vi "dual camera load displacement.vi"() -> ()   [LabVIEW 2013]
uses:
  <vilib>/userdefined/High Color/IMAQdx.ctl
  <vilib>/vision/driver/IMAQdx.llb/IMAQdx Buffer Number Mode.ctl
  <vilib>/Analysis/baseanly.llb/Mean (DBL).vi
  Instance           1 30Saved   Shear-C273-with-Unload .vi
  Instance           4 30Saved   Shear-C273-with-Unload .vi
  <vilib>/vision/driver/NI_Vision_Acquisition_Software.lvlib
  <resource>/objmgr/imaqdx.rc
  <vilib>/Analysis/NI_AALBase.lvlib
panel:
  in  "Shutter 3":dbl(slide)=20.0 min=0.0 max=4095.0 step=1.0 scale=4.095..4095.0 scale format="%#.0f"
  in  "Brightness 3":dbl(slide)=200.0 min=0.0 max=255.0 step=1.0 scale=0.0..255.0
  in  "Gain 3":dbl(slide)=702.0 min=350.0 max=1000.0 step=1.0 scale=350.0..1000.0
  out "Boolean 2":bool
  in  "Image Sampling Frequency (ms) 2":u32=100
  in  "Save nth image 2":i32=10
  in  "Capture Current Image 2":bool
  out "Diagonal":T1(plugin-control)
  in  "Video Mode Top 2":u32(ring)=47 items=["320x240 Color"=4, "640x480 Mono8"=9, "640x480 Mono16"=19, "640x480 Color"=14, "800x600 Mono8"=21, "800x600 Mono16"=27, "800x600 Color"=24, "1024x768 Mono8"=30, "1024x768 Mono16"=36, "1024x768 Color"=33, "1280x960 Mono8"=40, "1280x960 Mono16"=46, "1280x960 Color"=43, "1388x1038 Color"=47, "1388x1038 Mono"=48]
  in  "Session In Top View 2":T2="cam1"
  out "Side":T1(plugin-control)
  out "x-y":u32
  out "Boolean":bool
  in  "Begin Loading 2":bool
  in  "Shutter":dbl(slide)=20.0 min=0.0 max=4095.0 step=1.0 scale=4.095..4095.0 scale format="%#.0f"
  in  "Brightness":dbl(slide)=200.0 min=0.0 max=255.0 step=1.0 scale=0.0..255.0
  in  "Gain":dbl(slide)=702.0 min=350.0 max=1000.0 step=1.0 scale=350.0..1000.0
  in  "Video Mode Top":u32(ring)=47 items=["320x240 Color"=4, "640x480 Mono8"=9, "640x480 Mono16"=19, "640x480 Color"=14, "800x600 Mono8"=21, "800x600 Mono16"=27, "800x600 Color"=24, "1024x768 Mono8"=30, "1024x768 Mono16"=36, "1024x768 Color"=33, "1280x960 Mono8"=40, "1280x960 Mono16"=46, "1280x960 Color"=43, "1388x1038 Color"=47, "1388x1038 Mono"=48]
  in  "Session In Top View":T2="cam1"
  in  "Image Sampling Frequency (ms)":u32=100
  in  "Stop 2":bool
  in  "Save nth image":i32=10
  in  "Capture Current Image":bool
  in  "Begin Loading":bool
  out "Displacement (mm)":dbl
  in  "Pause":bool
  out "Crosshead Displacement":cluster{dbl[], dbl[]}(graph)
  in  "Unload Velocity":dbl=500.0
  in  "Unload":bool
  in  "Load Cell\nSelection":enum16{"300lb", "5lb", "50lb", "100lb"}(ring)=enum."50lb"
  in  "Distance to Travel (microns) \nup is positive":dbl=250000.0
  in  "Velocity (microns/sec)":dbl=5.0
  in  "Filename":string="test2"
  in  "Storage Directory":path=path "C:/Documents and Settings/AMS_Beckman/My Documents/Users_2010_2011/Jason_Patrick"
  in  "Material":string
  in  "Stop":bool
  # "Edge Parameters"
  # "Top View Camera"
types:
  T1 = typedef "IMAQ Image.ctl" = refnum<image>
  T2 = typedef "IMAQdx.ctl" = refnum<k21>
  T3 = typedef "Image Type" = u32
  T4 = enum16{"open", "open or create", "create or replace", "create", "open (read only)"}
  T5 = typedef "NI_Vision_Acquisition_Software.lvlib/IMAQdx Buffer Number Mode.ctl" = enum32{"Next", "Last", "Buffer Number"}
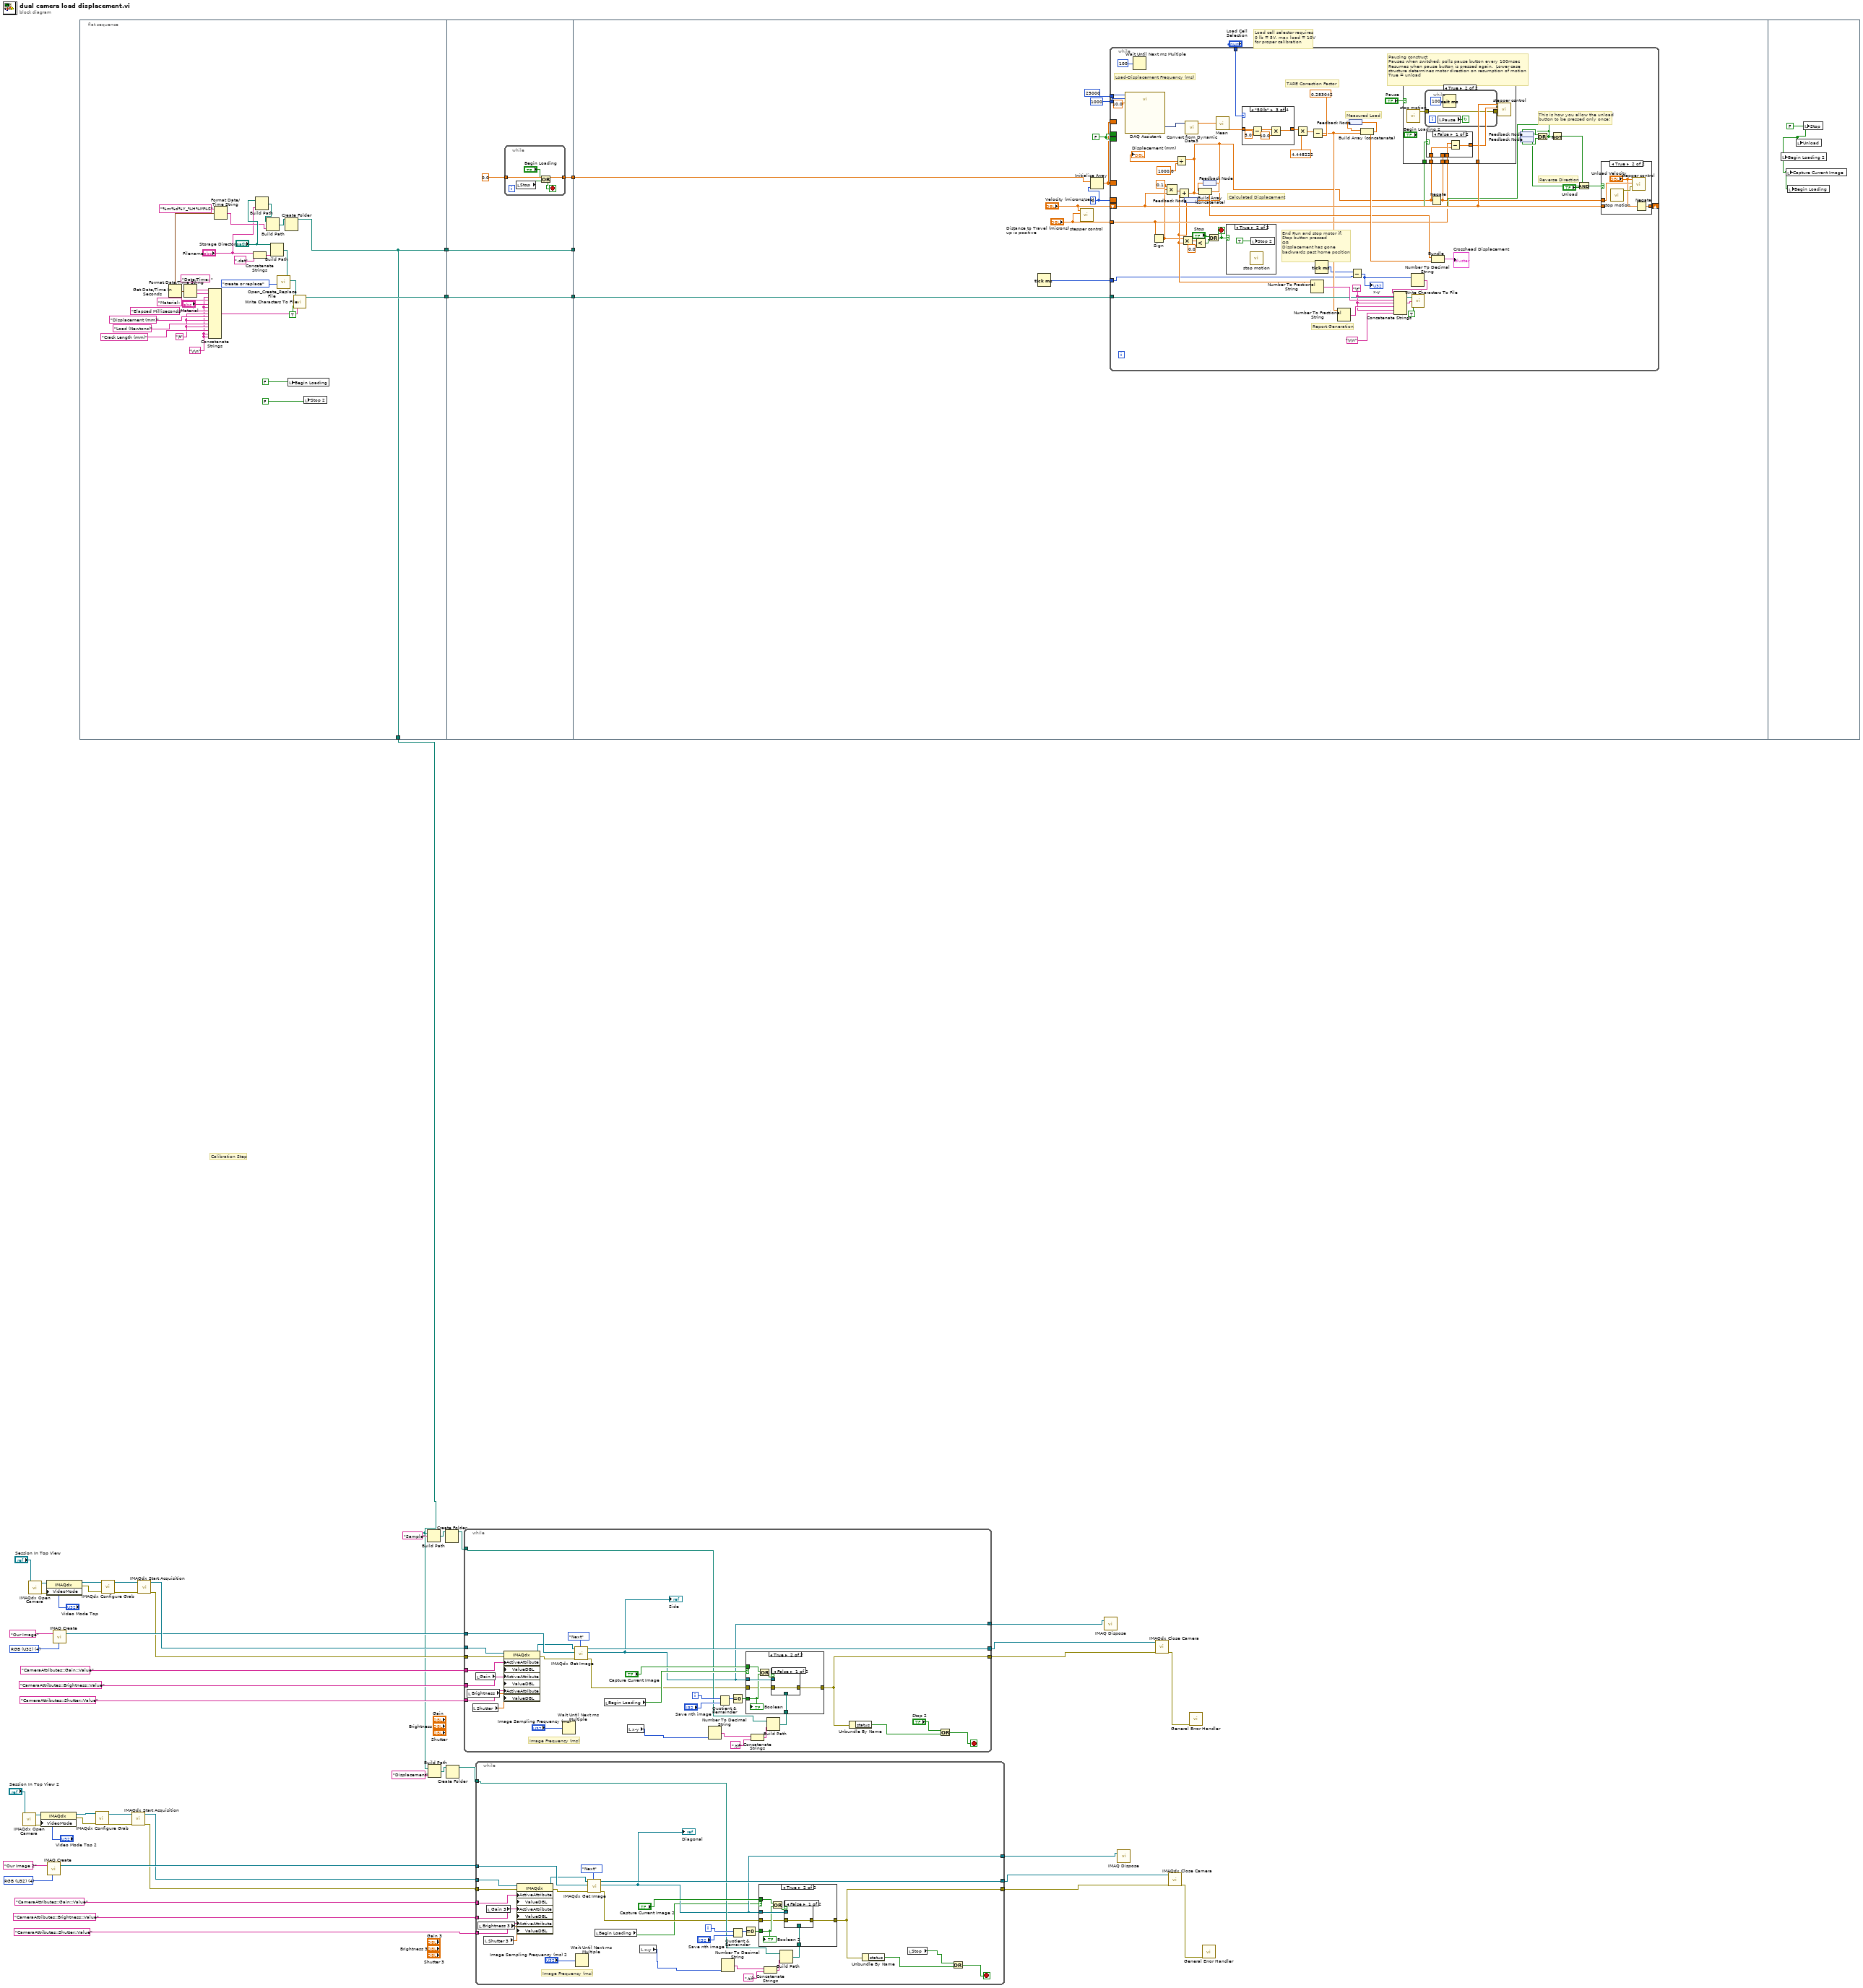
[diagram p0: block diagram]
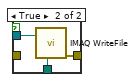
[diagram p3: hidden frame]
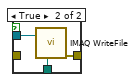
[diagram p5: hidden frame]
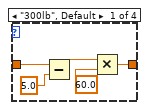
[diagram p10: hidden frame]
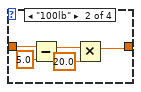
[diagram p11: hidden frame]
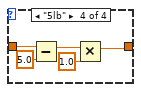
[diagram p12: hidden frame]
diagram:
  w23 = T3 4 items=["Grayscale (U8)", "Grayscale (I16)", "Grayscale (SGL)", "Complex (CSG)", "RGB (U32)", "HSL (U32)", "RGB (U64)"] ("Image Type")
  w43 = T3 4 items=["Grayscale (U8)", "Grayscale (I16)", "Grayscale (SGL)", "Complex (CSG)", "RGB (U32)", "HSL (U32)", "RGB (U64)"] ("Image Type")
  # "Calibration Step"
  n1 = call <vilib>:"IMAQdx Open Camera.vi"("Session In"="Session In Top View 2") -> ("error out"=w21:errorcluster, "Session Out"=w22:T2)  [unwired: 9 in]
  n2 = call <vilib>:"IMAQdx Open Camera.vi"("Session In"="Session In Top View") -> ("error out"=w41:errorcluster, "Session Out"=w42:T2)  [unwired: 9 in]
  n3 = property class="IMAQdx"(reference=w22, error in=w21, "VideoMode"="Video Mode Top 2") -> (reference out=w19:T2, error out=w20:errorcluster)
  n4 = property class="IMAQdx"(reference=w42, error in=w41, "VideoMode"="Video Mode Top") -> (reference out=w39:T2, error out=w40:errorcluster)
  n5 = call "IMAQ Create"("Image Name"="Our Image 2", "Image Type"=w23) -> ("New Image"=w10:T1)  [unwired: 3 in, 1 out]
  n6 = call "IMAQ Create"("Image Name"="Our Image", "Image Type"=w43) -> ("New Image"=w34:T1)  [unwired: 3 in, 1 out]
  n7 = flat-sequence {
    tunnel: [w71] -> w52
    tunnel: [w65] -> w50
    tunnel: [w65] -> w2
    tunnel: w52 -> [w84]
    tunnel: [w84] -> w51
    tunnel: w50 -> [w83]
    tunnel: [w83] -> w49
    tunnel: [w81] -> w48
    tunnel: w51 -> [w94]
    tunnel: w49 -> [_]
    tunnel: w48 -> [w90]
    frame #0 {
      w58 = "\t"
      w57 = "\r\n"
      n8 = Get Date/Time In Seconds() -> (seconds since 1Jan1904=w67:timestamp)
      n9 = Format Date/Time String(seconds (now)=w67) -> (date/time string=w73:string)  [unwired: 2 in]
      n10 = Concatenate Strings("Date/Time: ", w73, w57, "Material:  ", "Material", w57, "Elapsed Milliseconds" ("string"), w58, "Displacement (mm)" ("string"), w58, "Load (Newtons)" ("string"), w58, "Crack Length (mm)" ("string"), w57, w57) -> (w75:string)
      n11 = Format Date/Time String(time format string (%c)="%m%d%Y_%H%M%S", seconds (now)=w67) -> (date/time string=w54:string)  [unwired: 1 in]
      n12 = Concatenate Strings("Filename", ".dat") -> (w77:string)
      n13 = Build Path(base path="Storage Directory", name or relative path="Filename") -> (appended path=w55:path)
      n14 = Build Path(base path=w55, name or relative path=w54) -> (appended path=w69:path)
      n15 = Build Path(base path="Storage Directory", name or relative path=w77) -> (appended path=w70:path)
      n16 = call <vilib>:"Open_Create_Replace File.vi"("function (open:0)"=T4."create or replace", "file path"=w70) -> ("new file path"=w79:path)  [unwired: 6 in, 3 out]
      n17 = Create Folder(path (use dialog)=w69) -> (created path=w65:path)  [unwired: 2 in, 2 out]
      n18 = local write "Begin Loading"(FALSE ("Begin Loading")) -> ()
      n19 = call <vilib>:"Write Characters To File.vi"("append to file? (new file:F)"=TRUE, "character string"=w75, "file path (dialog if empty)"=w79) -> ("new file path (Not A Path if cancelled)"=w71:path)  [unwired: 2 in]
      n20 = local write "Stop 2"(FALSE ("Stop 2")) -> ()
    }
    frame #1 {
      n21 = while {
        tunnel: [w88] -> w81
        tunnel: 0.0 ("element") -> [w88]
        stop <- w86 stop-if-true
        n22 = local read "Stop"() -> (w85:bool)
        n23 = Or(x="Begin Loading", y=w85) -> (x .or. y?=w86:bool)
      }
    }
    frame #2 {
      w99 = FALSE
      w98 = 0 ("dimension size")
      # "Load cell selector requires\n0 lb = 5V, max load = 10V\nfor proper calibration"
      n24 = Tick Count (ms)() -> (millisecond timer value=w89:u32)
      n25 = call "stepper control.vi"("Distance to Travel (microns) \nup  is positive"="Distance to Travel (microns) \nup is positive", "Velocity (microns/sec)"="Velocity (microns/sec)") -> ()  [unwired: 9 in, 1 out]
      n26 = Initialize Array(w90, w98) -> (w97:dbl[])
      n27 = while {
        tunnel: "Load Cell\nSelection" -> [w150]
        tunnel: w94 -> [w140]
        shift-right: [w139] -> _
        shift-left: "Velocity (microns/sec)" -> [w124]
        tunnel: "Distance to Travel (microns) \nup is positive" -> [w121]
        border: w97 -> [_]
        border: w98 -> [_]
        border: w97 -> [_]
        border: w99 -> [_]
        border: w99 -> [_]
        tunnel: 25000 ("Sampling Rate") -> [w115]
        tunnel: 1000 ("Sampling Rate") -> [w114]
        tunnel: w89 -> [w103]
        stop <- w138 stop-if-true
        w105 = "\t"
        # "Load-Displacement Frequency (ms)"
        # "TARE Correction Factor"
        # "Pausing construct\nPauses when switched; polls pause button every 100msec\nResumes when pause button is pressed again.  Lower case\nstructure determines motor direction on resumption of motion\nTrue = unload"
        # "This is how you allow the unload\nbutton to be pressed only once!"
        # "Reverse Direction"
        # "Calculated Displacement"
        # "Measured Load"
        # "End Run and stop motor if:\nStop button pressed\nOR\nDisplacement has gone \nbackwards past home position"
        # "Report Generation"
        n28 = call "DAQ Assistant"("rate"=w115, "number of samples"=w114, "timeout (s)"=10.0 ("timeout (sec)")) -> ("data"=w116:dynamicdata)  [unwired: 14 in, 2 out]
        n29 = Wait Until Next ms Multiple(millisecond multiple=100 ("Loop Timing")) -> ()  [unwired: 1 out]
        n30 = Sign(1:w121) -> (0:w118:dbl)
        n31 = Compound Arithmetic op=MULTIPLY(0.1 ("x"), w118, w124) -> (w135:dbl)
        n32 = feedback #1() -> (w119:dbl)
        n33 = Add(x=w135, y=w119) -> (x+y=w108:dbl)
        n34 = Divide(x=w108, y=1000.0 ("timeout (sec)")) -> (x/y=→"Displacement (mm)":dbl)
        n35 = Multiply(x=w118, y=w119) -> (x*y=w120:dbl)
        n36 = feedback-in #1(w108) -> ()
        n37 = call "Convert from Dynamic Data3"("Dynamic Data Type"=w116) -> ("Array"=w113:dbl[])  [unwired: 3 in]
        n38 = Less?(x=w120, y=0.0) -> (x < y?=w137:bool)
        n39 = feedback #2() -> (w146:dbl[])
        n40 = Build Array (concatenate)(w146, w108) -> (w126:dbl[])
        n41 = feedback-in #2(w126) -> ()
        n42 = Or(x="Stop", y=w137) -> (x .or. y?=w138:bool)
        n43 = call-poly <vilib>:"Mean.vi"("X"=w113) -> ("mean"=w112:dbl)  [unwired: 1 out]
        n44 = case shown="True" w138 {
          frame False {
          }
          frame True {
            n45 = call "stop motion.vi"() -> ()  [unwired: 11 in, 1 out]
            n46 = local write "Stop 2"(TRUE ("Stop 2")) -> ()
          }
        }
        n47 = case shown="\"50lb\"" w150 {
          tunnel: w112 -> [w175 w179 w187 w192]
          tunnel: [w177 w178 w186 w191] -> w148
          frame "300lb", Default {
            n48 = Subtract(x=w175, y=5.0) -> (x-y=w173:dbl)
            n49 = Multiply(x=w173, y=60.0) -> (x*y=w177:dbl)
          }
          frame "100lb" {
            n50 = Subtract(x=w179, y=5.0) -> (x-y=w181:dbl)
            n51 = Multiply(x=w181, y=20.0) -> (x*y=w178:dbl)
          }
          frame "50lb" {
            n52 = Subtract(x=w187, y=5.0) -> (x-y=w184:dbl)
            n53 = Multiply(x=w184, y=10.0) -> (x*y=w186:dbl)
          }
          frame "5lb" {
            n54 = Subtract(x=w192, y=5.0) -> (x-y=w189:dbl)
            n55 = Multiply(x=w189, y=1.0) -> (x*y=w191:dbl)
          }
        }
        n56 = Multiply(x=w148, y=4.448222) -> (x*y=w111:dbl)
        n57 = Number To Fractional String(number=w119) -> (F-format string=w142:string)  [unwired: 3 in]
        n58 = Subtract(x=w111, y=0.283042) -> (x-y=w109:dbl)
        n59 = Tick Count (ms)() -> (millisecond timer value=w102:u32)
        n60 = Number To Fractional String(number=w109) -> (F-format string=w141:string)  [unwired: 3 in]
        n61 = feedback #3() -> (w147:dbl[])
        n62 = Subtract(x=w102, y=w103) -> (x-y=w101:u32)
        "x-y" <- w101
        n63 = Build Array (concatenate)(w147, w109) -> (w127:dbl[])
        n64 = feedback-in #3(w127) -> ()
        n65 = Number To Decimal String(number=w101) -> (decimal integer string=w104:string)  [unwired: 1 in]
        n66 = Concatenate Strings(w104, w105, w142, w105, w141, w105, "\r\n") -> (w144:string)
        n67 = call <vilib>:"Write Characters To File.vi"("append to file? (new file:F)"=TRUE, "character string"=w144, "file path (dialog if empty)"=w140) -> ()  [unwired: 2 in, 1 out]
        n68 = Negate(x=w108) -> (-x=w122:dbl)
        n69 = Bundle(w126, w127) -> (→"Crosshead Displacement":cluster{dbl[], dbl[]})  [unwired: 1 in]
        n70 = feedback #4() -> (w134:bool)
        n71 = feedback #5() -> (w132:bool)
        n72 = Or(x=w134, y=w132) -> (x .or. y?=w123:bool)
        n73 = case shown="True" "Pause" {
          tunnel: w124 -> [_ w157]
          tunnel: w123 -> [_ w156]
          tunnel: w122 -> [_ w155]
          tunnel: w121 -> [_ w154]
          tunnel: w108 -> [_ w152]
          frame False {
          }
          frame True {
            n74 = call "stop motion.vi"() -> ("error out"=w159:errorcluster)  [unwired: 11 in]
            n75 = while {
              tunnel: [w164] -> w158
              tunnel: w159 -> [w164]
              stop <- w166 continue-if-true
              n76 = local read "Pause"() -> (w166:bool)
              n77 = Wait (ms)(milliseconds to wait=100 ("Loop Timing")) -> ()  [unwired: 1 out]
            }
            n78 = case shown="False" w156 {
              tunnel: w155 -> [_ w163]
              tunnel: w154 -> [w161 _]
              tunnel: [w162 w163] -> w153
              tunnel: w152 -> [w160 _]
              frame False {
                n79 = Subtract(x=w161, y=w160) -> (x-y=w162:dbl)
              }
              frame True {
              }
            }
            n80 = call "stepper control.vi"("error in (no error)"=w158, "Distance to Travel (microns) \nup  is positive"=w153, "Velocity (microns/sec)"=w157) -> ()  [unwired: 8 in, 1 out]
          }
        }
        n81 = feedback-in #4(w123) -> ()
        n82 = Not(x=w123) -> (.not. x?=w133:bool)
        n83 = And(x=w133, y="Unload") -> (x .and. y?=w130:bool)
        n84 = feedback-in #5(w130) -> ()
        n85 = case shown="True" w130 {
          tunnel: w122 -> [_ w170]
          tunnel: [w167 w169] -> w139
          tunnel: w124 -> [w167 _]
          frame False {
          }
          frame True {
            n86 = call "stop motion.vi"() -> ("error out"=w171:errorcluster)  [unwired: 11 in]
            n87 = call "stepper control.vi"("error in (no error)"=w171, "Distance to Travel (microns) \nup  is positive"=w170, "Velocity (microns/sec)"="Unload Velocity") -> ()  [unwired: 8 in, 1 out]
            n88 = Negate(x="Unload Velocity") -> (-x=w169:dbl)
          }
        }
      }
    }
    frame #3 {
      w193 = FALSE ("Stop")
      n89 = local write "Begin Loading 2"(w193) -> ()
      n90 = local write "Capture Current Image"(w193) -> ()
      n91 = local write "Begin Loading"(w193) -> ()
      n92 = local write "Unload"(w193) -> ()
      n93 = local write "Stop"(w193) -> ()
    }
  }
  n94 = call <vilib>:"IMAQdx Configure Grab.vi"("error in"=w20, "Session In"=w19) -> ("error out"=w17:errorcluster, "Session Out"=w18:T2)  [unwired: 8 in]
  n95 = call <vilib>:"IMAQdx Configure Grab.vi"("error in"=w40, "Session In"=w39) -> ("error out"=w37:errorcluster, "Session Out"=w38:T2)  [unwired: 8 in]
  n96 = call <vilib>:"IMAQdx Start Acquisition.vi"("error in"=w17, "Session In"=w18) -> ("error out"=w8:errorcluster, "Session Out"=w9:T2)  [unwired: 8 in]
  n97 = call <vilib>:"IMAQdx Start Acquisition.vi"("error in"=w37, "Session In"=w38) -> ("error out"=w25:errorcluster, "Session Out"=w35:T2)  [unwired: 8 in]
  n98 = Build Path(base path=w2, name or relative path="Sample") -> (appended path=w27:path)
  n99 = Build Path(base path=w2, name or relative path="Displacement") -> (appended path=w4:path)
  n100 = Create Folder(path (use dialog)=w27) -> (created path=w26:path)  [unwired: 2 in, 2 out]
  n101 = Create Folder(path (use dialog)=w4) -> (created path=w3:path)  [unwired: 2 in, 2 out]
  n102 = while {
    tunnel: w34 -> [w219]
    tunnel: "CameraAttributes::Gain::Value" ("ActiveAttribute") -> [w225]
    tunnel: "CameraAttributes::Brightness::Value" ("ActiveAttribute") -> [w224]
    tunnel: "CameraAttributes::Shutter::Value" ("ActiveAttribute") -> [w223]
    tunnel: [w213] -> w47
    tunnel: w25 -> [w217]
    tunnel: [w210] -> w46
    tunnel: w35 -> [w214]
    tunnel: [w194] -> w29
    tunnel: w26 -> [w196]
    i -> [w206]
    stop <- w209 stop-if-true
    # "Image Frequency (ms)"
    n103 = local read "Brightness"() -> (w221:dbl)
    n104 = local read "Shutter"() -> (w220:dbl)
    n105 = local read "Gain"() -> (w222:dbl)
    n106 = property class="IMAQdx"(reference=w214, error in=w217, "ActiveAttribute"=w225, "ValueDBL"=w222, "ActiveAttribute"=w224, "ValueDBL"=w221, "ActiveAttribute"=w223, "ValueDBL"=w220) -> (reference out=w216:T2, error out=w215:errorcluster)
    n107 = Wait Until Next ms Multiple(millisecond multiple="Image Sampling Frequency (ms)") -> ()  [unwired: 1 out]
    n108 = call <vilib>:"IMAQdx Get Image.vi"("Buffer Number Mode (Next)"=IMAQdx_Buffer_Number_Mode."Next", "error in"=w215, "Image In"=w219, "Session In"=w216) -> ("error out"=w195:errorcluster, "Image Out"=w194:T1, "Session Out"=w213:T2)  [unwired: 4 in, 1 out]
    "Side" <- w194
    n109 = local read "Begin Loading"() -> (w202:bool)
    n110 = local read "x-y"() -> (w199:u32)
    n111 = Number To Decimal String(number=w199) -> (decimal integer string=w197:string)  [unwired: 1 in]
    n112 = Quotient & Remainder(x=w206, y="Save nth image") -> (x-y*floor(x/y)=w204:i32)  [unwired: 1 out]
    n113 = Equal To 0?(x=w204) -> (x = 0?=w203:bool)
    n114 = Concatenate Strings(w197, ".tif") -> (w211:string)
    n115 = Build Path(base path=w196, name or relative path=w211) -> (appended path=w212:path)
    n116 = case shown="True" w202 {
      tunnel: w194 -> [_ w233]
      tunnel: w212 -> [_ w231]
      tunnel: [w226 w232] -> w210
      tunnel: "Capture Current Image" -> [_ w229]
      tunnel: w203 -> [_ w228]
      tunnel: w195 -> [w226 w227]
      frame False {
      }
      frame True {
        n117 = Or(x=w229, y=w228) -> (x .or. y?=w230:bool)
        n118 = case shown="False" w230 {
          tunnel: w233 -> [_ w237]
          tunnel: [w234 w236] -> w232
          tunnel: w231 -> [_ w235]
          tunnel: w227 -> [w234 _]
          frame False {
          }
          frame True {
            n119 = call "IMAQ WriteFile"("File Path"=w235, "Image"=w237) -> ("error out"=w236:errorcluster)  [unwired: 6 in]
          }
        }
        "Boolean" <- w228
      }
    }
    n120 = Unbundle By Name(w210) -> ("status"=w208:bool)
    n121 = Or(x="Stop 2", y=w208) -> (x .or. y?=w209:bool)
  }
  n122 = while {
    tunnel: w10 -> [w263]
    tunnel: "CameraAttributes::Gain::Value" ("ActiveAttribute") -> [w269]
    tunnel: "CameraAttributes::Brightness::Value" ("ActiveAttribute") -> [w268]
    tunnel: "CameraAttributes::Shutter::Value" ("ActiveAttribute") -> [w267]
    tunnel: [w257] -> w14
    tunnel: w8 -> [w261]
    tunnel: [w254] -> w13
    tunnel: w9 -> [w258]
    tunnel: [w241] -> w11
    tunnel: w3 -> [w243]
    i -> [w250]
    stop <- w253 stop-if-true
    # "Image Frequency (ms)"
    n123 = local read "Brightness 3"() -> (w265:dbl)
    n124 = local read "Shutter 3"() -> (w264:dbl)
    n125 = local read "Gain 3"() -> (w266:dbl)
    n126 = property class="IMAQdx"(reference=w258, error in=w261, "ActiveAttribute"=w269, "ValueDBL"=w266, "ActiveAttribute"=w268, "ValueDBL"=w265, "ActiveAttribute"=w267, "ValueDBL"=w264) -> (reference out=w260:T2, error out=w259:errorcluster)
    n127 = Wait Until Next ms Multiple(millisecond multiple="Image Sampling Frequency (ms) 2") -> ()  [unwired: 1 out]
    n128 = call <vilib>:"IMAQdx Get Image.vi"("Buffer Number Mode (Next)"=IMAQdx_Buffer_Number_Mode."Next", "error in"=w259, "Image In"=w263, "Session In"=w260) -> ("error out"=w242:errorcluster, "Image Out"=w241:T1, "Session Out"=w257:T2)  [unwired: 4 in, 1 out]
    "Diagonal" <- w241
    n129 = local read "Begin Loading"() -> (w239:bool)
    n130 = local read "x-y"() -> (w238:u32)
    n131 = Number To Decimal String(number=w238) -> (decimal integer string=w244:string)  [unwired: 1 in]
    n132 = Quotient & Remainder(x=w250, y="Save nth image 2") -> (x-y*floor(x/y)=w248:i32)  [unwired: 1 out]
    n133 = Equal To 0?(x=w248) -> (x = 0?=w247:bool)
    n134 = Concatenate Strings(w244, ".tif") -> (w255:string)
    n135 = Build Path(base path=w243, name or relative path=w255) -> (appended path=w256:path)
    n136 = case shown="True" w239 {
      tunnel: w241 -> [_ w277]
      tunnel: w256 -> [_ w275]
      tunnel: [w270 w276] -> w254
      tunnel: "Capture Current Image 2" -> [_ w273]
      tunnel: w247 -> [_ w272]
      tunnel: w242 -> [w270 w271]
      frame False {
      }
      frame True {
        n137 = Or(x=w273, y=w272) -> (x .or. y?=w274:bool)
        n138 = case shown="False" w274 {
          tunnel: w277 -> [_ w281]
          tunnel: [w278 w280] -> w276
          tunnel: w275 -> [_ w279]
          tunnel: w271 -> [w278 _]
          frame False {
          }
          frame True {
            n139 = call "IMAQ WriteFile"("File Path"=w279, "Image"=w281) -> ("error out"=w280:errorcluster)  [unwired: 6 in]
          }
        }
        "Boolean 2" <- w272
      }
    }
    n140 = Unbundle By Name(w254) -> ("status"=w252:bool)
    n141 = local read "Stop"() -> (w240:bool)
    n142 = Or(x=w240, y=w252) -> (x .or. y?=w253:bool)
  }
  n143 = call "IMAQ Dispose"("Image"=w29) -> ()  [unwired: 5 in, 1 out]
  n144 = call "IMAQ Dispose"("Image"=w11) -> ()  [unwired: 5 in, 1 out]
  n145 = call <vilib>:"IMAQdx Close Camera.vi"("error in"=w46, "Session In"=w47) -> ("error out"=w45:errorcluster)  [unwired: 9 in]
  n146 = call <vilib>:"IMAQdx Close Camera.vi"("error in"=w13, "Session In"=w14) -> ("error out"=w12:errorcluster)  [unwired: 9 in]
  n147 = call <vilib>:"General Error Handler.vi"("error in (no error)"=w45) -> ()  [unwired: 10 in, 5 out]
  n148 = call <vilib>:"General Error Handler.vi"("error in (no error)"=w12) -> ()  [unwired: 10 in, 5 out]
